vi "msgMatch.vi"(8 "errorIn":errorcluster, 10 "msgMatcher":string, 11 "refer":refnum<queue>) -> (0 "errorOut":errorcluster, 2 "match":bool, 3 "refer":refnum<queue>)   [LabVIEW 2017]
doc: "refer：消息队列\nmsgMatcher：消息匹配通配符\nmatch：是否匹配到消息"
uses:
  models/EMSGData.ctl
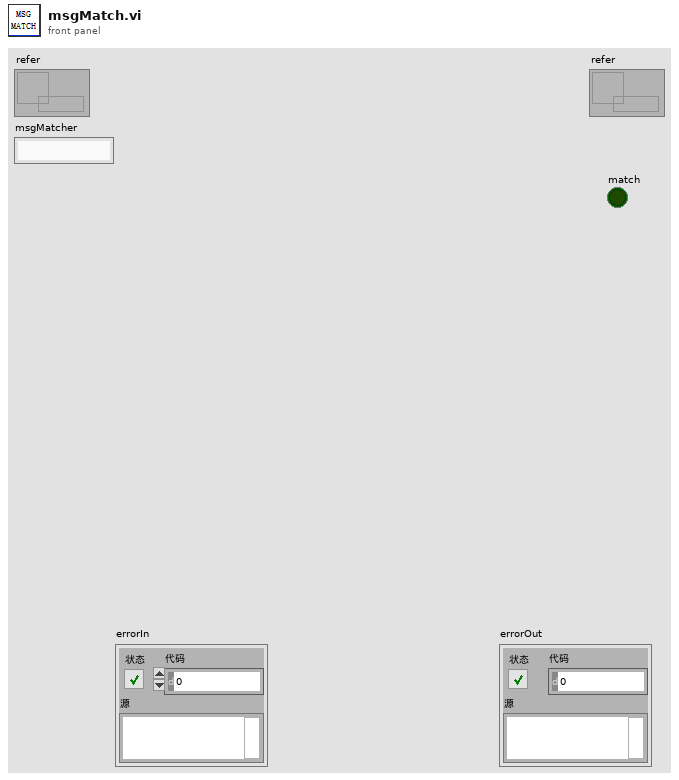
[diagram p1: front panel]
types:
  T1 = typedef "EMSGData.ctl" = cluster{"to":string, "from":string, "data":variant, "remark1":string, "remark 2":string}
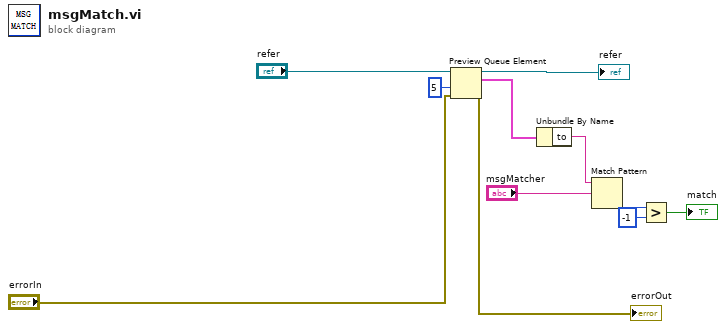
[diagram p0: block diagram]
diagram:
  n1 = Preview Queue Element(queue="refer", timeout in ms (-1)=5 ("超时毫秒(-1)"), error in (no error)="errorIn") -> (queue out=→"refer":refnum<queue>, element=w9:T1, error out=→"errorOut":errorcluster)  [unwired: 1 out]
  n2 = Unbundle By Name(w9) -> ("to"=w8:string)
  n3 = Match Pattern(string=w8, regular expression="msgMatcher") -> (offset past match=w6:i32)  [unwired: 1 in, 3 out]
  n4 = Greater?(x=w6, y=-1) -> (0:→"match":bool)
